vi "Fuente Programable.vi"() -> ()   [LabVIEW 2014]
panel:
  out "Waveform Chart":dbl(graph)
  in  "Set Point":dbl(slide) scale=0.0..5.0
  in  "VISA resource name":refnum<visa-resource-name>
  in  "stop":bool
  in  "Velocidad de Conexion":enum16{"115200", "9600"}(ring)
  in  "error in (no error)":errorcluster
  # "Puerto de Com. Serial Elegido"
  # "Velocidad de Conexion"
  # "Punto de Consigna (V)"
  # "Control de Error de Entrada"
  # "Constante derivativa"
  # "Constante Integral"
  # "Constante Proporcional"
  # "Detener Ejecucion"
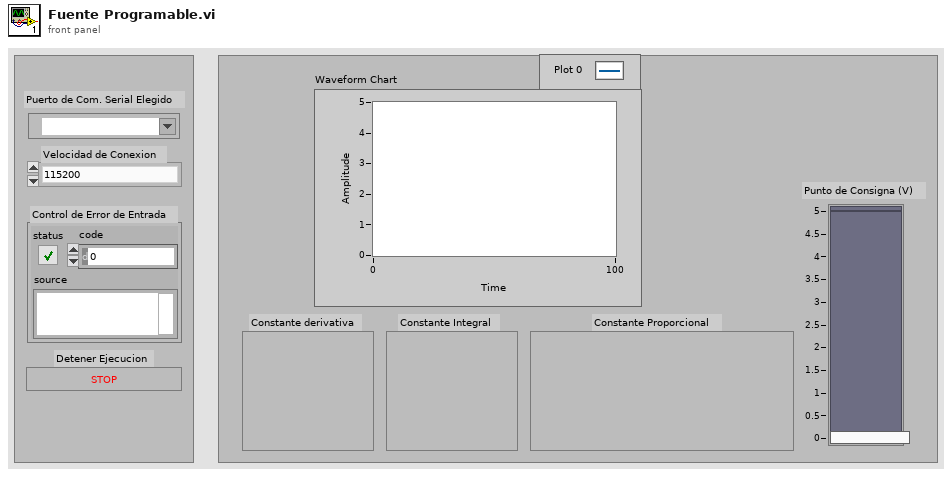
[diagram p1: front panel]
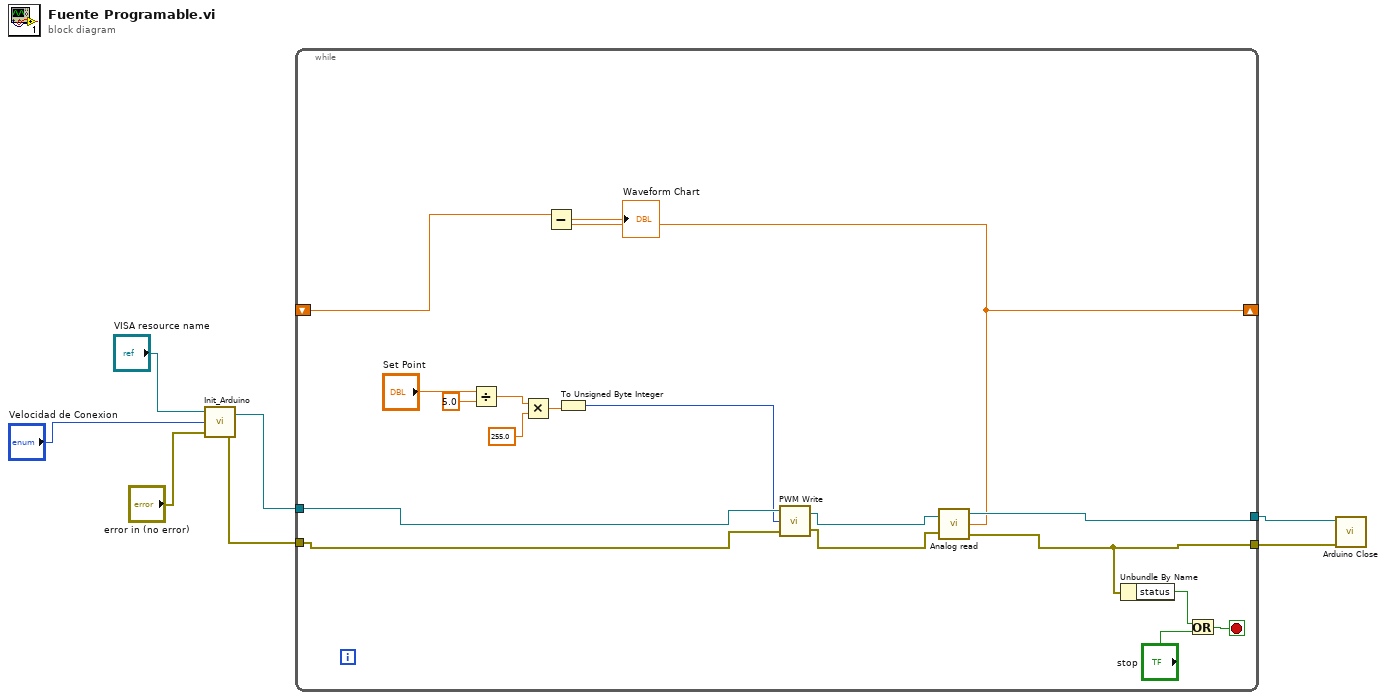
[diagram p0: block diagram]
diagram:
  n1 = call "Init_Arduino.vi"("error in (no error)"="error in (no error)", "Velocidad de Conexion"="Velocidad de Conexion", "VISA Refnum in"="VISA resource name") -> ("error out"=w3:errorcluster, "VISA Refnum out"=w5:refnum<visa-resource-name>)
  n2 = while {
    tunnel: w3 -> [w24]
    tunnel: w5 -> [w25]
    tunnel: [w19] -> w1
    tunnel: [w20] -> w2
    shift-right: [w16] -> _
    shift-left: _ -> [w15]
    stop <- w21 stop-if-true
    n3 = Divide(x="Set Point", y=5.0) -> (x/y=w11:dbl)
    n4 = Multiply(x=w11, y=255.0) -> (x*y=w9:dbl)
    n5 = To Unsigned Byte Integer(number=w9) -> (unsigned 8bit integer=w8:u8)
    n6 = call "PWM Write.vi"("error in (no error)"=w24, "Ciclo de Trabajo"=w8, "VISA Refnum in"=w25) -> ("error out"=w17:errorcluster, "VISA Refnum out"=w18:refnum<visa-resource-name>)
    n7 = call "Analog read.vi"("VISA Refnum in"=w18, "error in (no error)"=w17) -> ("VISA Refnum out"=w19:refnum<visa-resource-name>, "Numeric"=w16:dbl, "error out"=w20:errorcluster)
    n8 = Subtract(x=w15, y=w16) -> (x-y=→"Waveform Chart":dbl)
    n9 = Unbundle By Name(w20) -> ("status"=w23:bool)
    n10 = Or(x=w23, y="stop") -> (x .or. y?=w21:bool)
  }
  n11 = call "Arduino Close.vi"("error in (no error)"=w2, "VISA Refnum in"=w1) -> ()  [unwired: 10 in]
